vi "Untitled 3 (SubVI).vi"(9 "Fuel Type":bool, 10 "Fuel (kg/s)":dbl, 11 "Primery Air (kg/s)":dbl) -> (3 "Stoic":dbl)   [LabVIEW 2019]
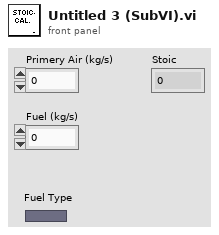
[diagram p1: front panel]
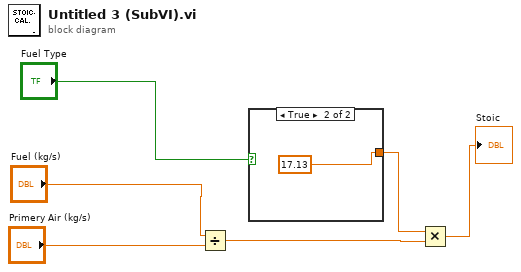
[diagram p0: block diagram]
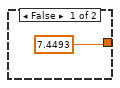
[diagram p2: hidden frame]
diagram:
  n1 = Divide(x="Fuel (kg/s)", y="Primery Air (kg/s)") -> (x/y=w4:dbl)
  n2 = case shown="True" "Fuel Type" {
    tunnel: [7.4493 17.13] -> w3
    frame False {
    }
    frame True {
    }
  }
  n3 = Multiply(x=w3, y=w4) -> (x*y=→"Stoic":dbl)
